vi "Say Hello.vi"(8 "error in (no error)":errorcluster, 11 "Test Instrument in":refnum<class "Test Instrument.lvclass">) -> (0 "error out":errorcluster, 3 "Test Instrument out":refnum<class "Test Instrument.lvclass">)   [LabVIEW 2020, in "Test.lvlib" / "Test Instrument.lvclass"]
uses:
  Test Instrument.lvclass
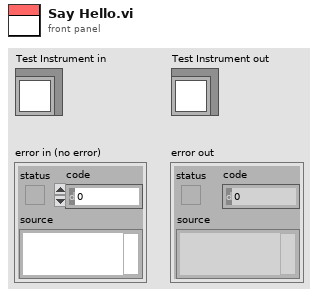
[diagram p1: front panel]
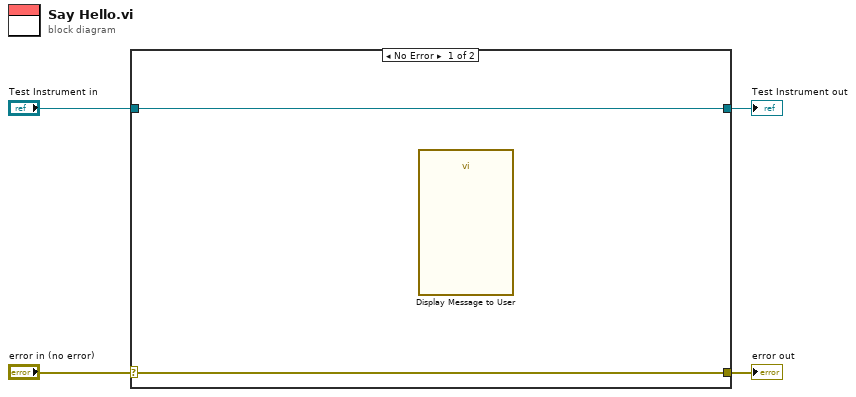
[diagram p0: block diagram]
diagram:
  n1 = case shown="No Error" "error in (no error)" {
    selector: "error in (no error)" -> [w5 w8]
    tunnel: [w5 w8] -> w3
    tunnel: [w6 w7] -> w1
    tunnel: "Test Instrument in" -> [w6 w7]
    frame No Error {
      n2 = call "Display Message to User"() -> ()  [unwired: 10 in, 2 out]
    }
    frame Error {
    }
  }
  "error out" <- w3
  "Test Instrument out" <- w1
